vi "Three Buttons Dialog Window.vi"(5 "Window Title":string, 6 "ESC =  Button 3 (T)":bool=TRUE, 7 "Return =  Button 1 (T)":bool=TRUE, 8 "Button 3 Text (Cancel)":string="Cancel", 9 "Button 2 Text":string="Other", 10 "Button 1 Text (OK)":string="OK", 11 "Message":string) -> (1 "3-button Dialog Output":T1=enum."Button 2")   [LabVIEW 2021]
uses:
  3-Button Dialog Output.ctl
  <vilib>/Utility/miscctls.llb/LVKeyTypeDef.ctl
panel:
  in  "Button 2":bool
  in  "Button 3":bool
  in  "Button 1":bool
  out "Displayed Message":string
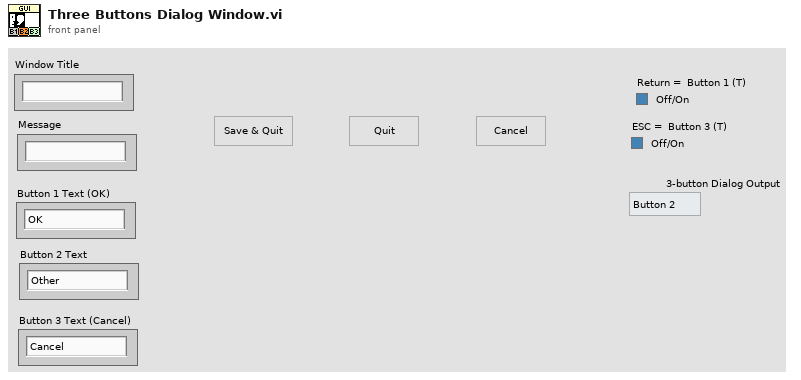
[diagram p1: front panel]
types:
  T1 = typedef "3-Button Dialog Output.ctl" = enum16{"Window Close", "Button 1", "Button 2", "Button 3"}
  T2 = typedef "LVKeyTypeDef.ctl" = cluster{"Focus":bool, "Control":bool, "Shift":bool, "Key":string}
  T3 = cluster{"Displayed Message":refnum<vi>, "Button 1":refnum<vi>, "Button 2":refnum<vi>, "Button 3":refnum<vi>}
  T4 = enum32{"Invalid", "Standard", "Closed", "Hidden", "Minimized", "Maximized"}
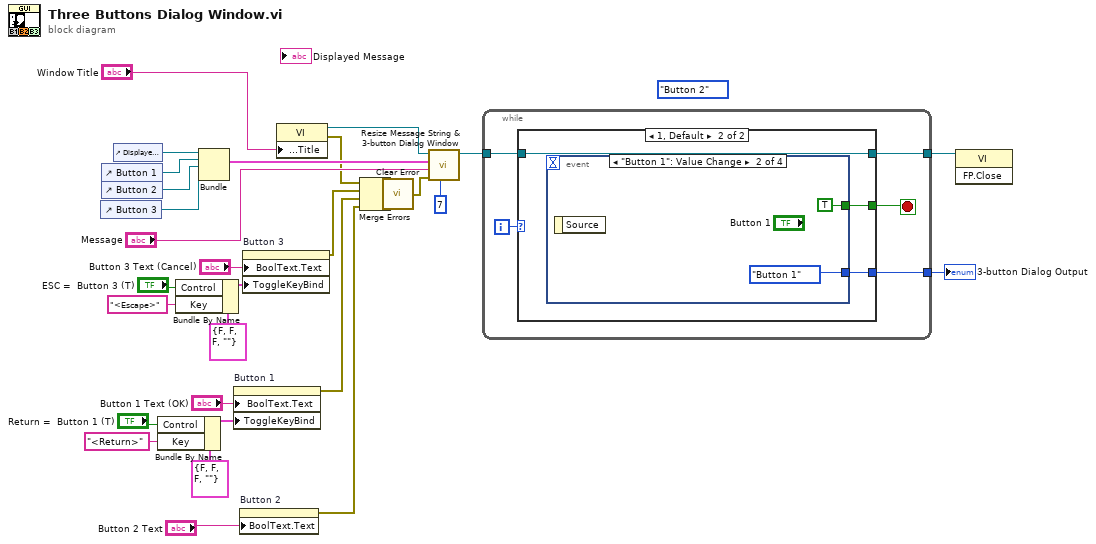
[diagram p0: block diagram]
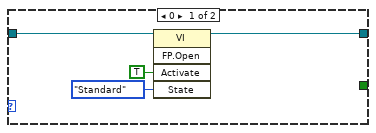
[diagram p2: hidden frame]
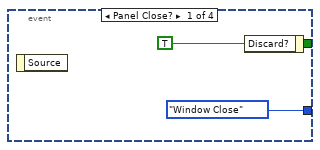
[diagram p3: hidden frame]
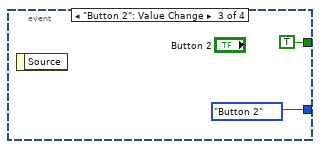
[diagram p4: hidden frame]
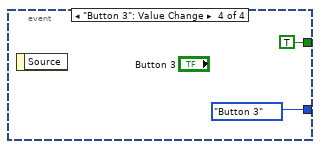
[diagram p5: hidden frame]
diagram:
  (unwired) 3-Button_Dialog_Output."Button 2" ("Justify Message (Left)")
  n1 = control-ref of="Button 3"() -> (w7:refnum<vi>)
  n2 = control-ref of="Button 1"() -> (w9:refnum<vi>)
  n3 = control-ref of="Button 2"() -> (w8:refnum<vi>)
  n4 = control-ref of="Displayed Message"() -> (w26:refnum<vi>)
  n5 = Bundle By Name(cluster=T2 {"Focus"=FALSE, "Control"=FALSE, "Shift"=FALSE, "Key"=""} ("Toggle Key Binding"), "Control"="Return =  Button 1 (T)", "Key"="<Return>") -> (w13:T2)
  n6 = Bundle By Name(cluster=T2 {"Focus"=FALSE, "Control"=FALSE, "Shift"=FALSE, "Key"=""} ("Toggle Key Binding"), "Control"="ESC =  Button 3 (T)", "Key"="<Escape>") -> (w18:T2)
  n7 = Bundle("Displayed Message"=w26, "Button 1"=w9, "Button 2"=w8, "Button 3"=w7) -> (w25:T3)  [unwired: 1 in]
  n8 = property on="Button 1" class="Bool"("BoolText.Text"="Button 1 Text (OK)", "ToggleKeyBind"=w13) -> (error out=w20:errorcluster)  [unwired: 2 in, 1 out]
  n9 = property on="Button 2" class="Bool"("BoolText.Text"="Button 2 Text") -> (error out=w5:errorcluster)  [unwired: 2 in, 1 out]
  n10 = property on="Button 3" class="Bool"("BoolText.Text"="Button 3 Text (Cancel)", "ToggleKeyBind"=w18) -> (error out=w22:errorcluster)  [unwired: 2 in, 1 out]
  n11 = property class="VI"("Front Panel.Title"="Window Title") -> (reference out=w4:refnum<vi>, error out=w3:errorcluster)  [unwired: 2 in]
  n12 = Merge Errors(w3, w22, w20, w5) -> (w21:errorcluster)
  n13 = call "Clear Error.vi"("Error In"=w21) -> ("no Error Out"=w11:errorcluster)  [unwired: 8 in]
  n14 = call "Resize Message String & 3-button Dialog Window.vi"("Max Number of Lines"=7, "Error In"=w11, "Message"="Message", "output Controls & Indicators"=w25, "VI Refnum"=w4) -> ("VI Refnum out"=w1:refnum<vi>)  [unwired: 5 in, 1 out]
  n15 = while {
    tunnel: w1 -> [w32]
    tunnel: [w31] -> w29
    tunnel: [w30] -> w6
    i -> [w33]
    stop <- w34 stop-if-true
    n16 = case shown="1, Default" w33 {
      tunnel: [_ w41] -> w34
      tunnel: w32 -> [w38 w40]
      tunnel: [w37 w40] -> w31
      tunnel: [_ w39] -> w30
      frame 0 {
        n17 = invoke class="VI" method="FP.Open"(reference=w38, "Activate"=TRUE ("Activate?"), "State"=T4."Standard") -> (reference out=w37:refnum<vi>)  [unwired: 2 in, 4 out]
      }
      frame 1, Default {
        n18 = event shown="[1] \"Button 1\": Value Change" {
          selector: _ -> [_ _ _ _]
          dyn-events: _ -> [_ _ _ _]
          timeout: _ -> [_ _ _ _]
          tunnel: [w43 TRUE ("Discard?") TRUE ("Discard?") TRUE ("Discard?")] -> w41
          tunnel: [3-Button_Dialog_Output."Window Close" ("3-button Dialog Output") 3-Button_Dialog_Output."Button 1" ("3-button Dialog Output") 3-Button_Dialog_Output."Button 2" ("3-button Dialog Output") 3-Button_Dialog_Output."Button 3" ("3-button Dialog Output")] -> w39
          event Panel Close? {
            w43 = TRUE ("Discard?")
            n19 = event-data() -> ()  [unwired: 1 in, 1 out]
            n20 = event-data("Discard?"=w43) -> ()  [unwired: 1 in, 1 out]
          }
          event "Button 1": Value Change {
            n21 = event-data() -> ()  [unwired: 1 in, 1 out]
          }
          event "Button 2": Value Change {
            n22 = event-data() -> ()  [unwired: 1 in, 1 out]
          }
          event "Button 3": Value Change {
            n23 = event-data() -> ()  [unwired: 1 in, 1 out]
          }
        }
      }
    }
  }
  "3-button Dialog Output" <- w6
  n24 = invoke class="VI" method="FP.Close"(reference=w29) -> ()  [unwired: 2 in, 3 out]
